vi "deltaGains.vi"(8 "Kp":dbl, 11 "e_psi":dbl) -> (0 "45degrees":bool, 2 "delta":dbl)   [LabVIEW 2014]
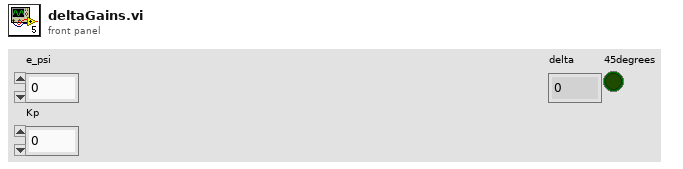
[diagram p1: front panel]
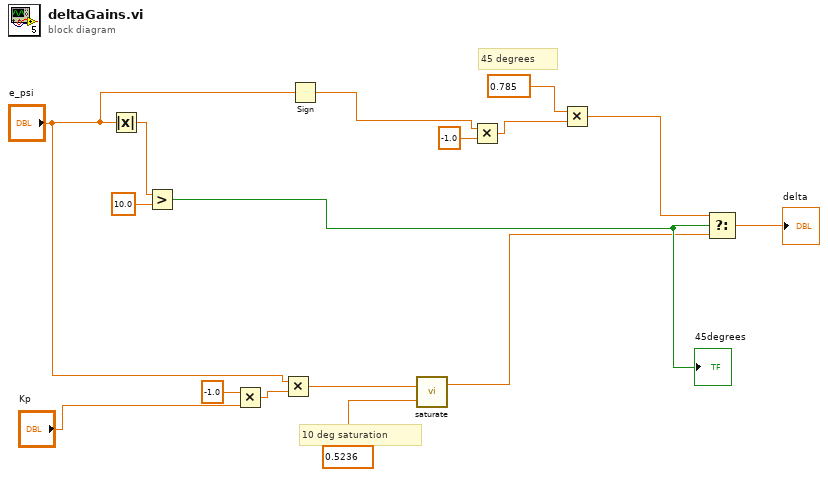
[diagram p0: block diagram]
diagram:
  # "45 degrees"
  # "10 deg saturation"
  n1 = Absolute Value(x="e_psi") -> (abs(x)=w10:dbl)
  n2 = Greater?(x=w10, y=10.0) -> (0:w12:bool)
  "45degrees" <- w12
  n3 = Multiply(x=-1.0, y="Kp") -> (x*y=w16:dbl)
  n4 = Multiply(x="e_psi", y=w16) -> (x*y=w9:dbl)
  n5 = Sign(1:"e_psi") -> (0:w3:dbl)
  n6 = call "saturate.vi"("amplitude"=0.5236, "value"=w9) -> ("saturated"=w8:dbl)  [unwired: 1 out]
  n7 = Multiply(x=w3, y=-1.0) -> (x*y=w1:dbl)
  n8 = Multiply(x=0.785 ("t"), y=w1) -> (x*y=w4:dbl)
  n9 = Select(t=w4, s=w12, f=w8) -> (s? t:f=→"delta":dbl)
